vi "Functional Test Prompt.vi"(10 "AutoAge.ini  File Path":path=path "\\\\Beco\\autoage/config/autoage.ini", 11 "System#":u8) -> ()   [LabVIEW 2021]
panel:
  in  "Rack":i8=1 min=1 max=16
  in  "Cancel":bool
  in  "OK":bool
  # "Run Functional Test on Rack ?"
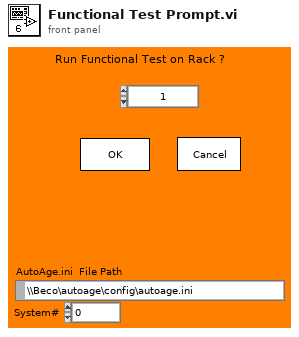
[diagram p1: front panel]
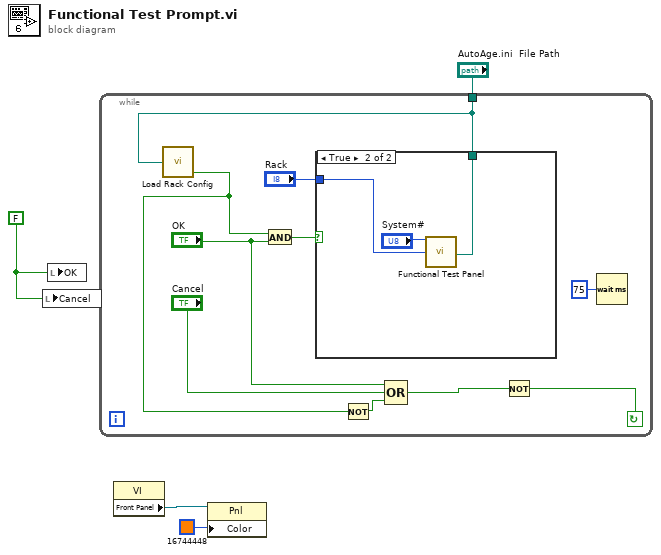
[diagram p0: block diagram]
diagram:
  w3 = FALSE ("OK")
  n1 = local write "Cancel"(w3) -> ()
  n2 = local write "OK"(w3) -> ()
  n3 = while {
    tunnel: "AutoAge.ini  File Path" -> [w9]
    stop <- w12 continue-if-true
    n4 = call "Load Rack Config"("AutoAge.ini  File Path"=w9) -> ("No Errors"=w5:bool)  [unwired: 2 out]
    n5 = And(x=w5, y="OK") -> (x .and. y?=w7:bool)
    n6 = case shown="True" w7 {
      tunnel: "Rack" -> [_ w15]
      tunnel: w9 -> [_ w17]
      frame False {
      }
      frame True {
        n7 = call "Functional Test Panel.vi"("System#"="System#", "Rack Number"=w15, "AutoAge.ini  File Path"=w17) -> ()  [unwired: 13 in]
      }
    }
    n8 = Not(x=w5) -> (.not. x?=w6:bool)
    n9 = Compound Arithmetic op=OR("OK", "Cancel", w6) -> (w13:bool)
    n10 = Not(x=w13) -> (.not. x?=w12:bool)
    n11 = Wait (ms)(milliseconds to wait=u32 75) -> ()  [unwired: 1 out]
  }
  n12 = property class="VI"() -> ("Front Panel"=w2:refnum<vi>)  [unwired: 2 in, 2 out]
  n13 = property class="Pnl"(reference=w2, "Color"=u32 16744448) -> ()  [unwired: 1 in, 2 out]
